vi "ObjectHandler.GetAllLogFiles.vi"(8 "error in (no error)":errorcluster, 11 "ObjectHandler in":refnum<class "ObjectHandler.lvclass">) -> (0 "error out":errorcluster, 1 "Found?":bool, 2 "Array":T1[](array[typedef]), 3 "ObjectHandler out":refnum<class "ObjectHandler.lvclass">)   [LabVIEW 2016, in "ObjectHandler.lvclass"]
uses:
  ObjectHandler.lvclass
  ObjectHandler.ObjectWType.ctl
  ObjectHandler.ObjectType.ctl
  ObjectHandler.lvclass/ObjectHandler.ctl
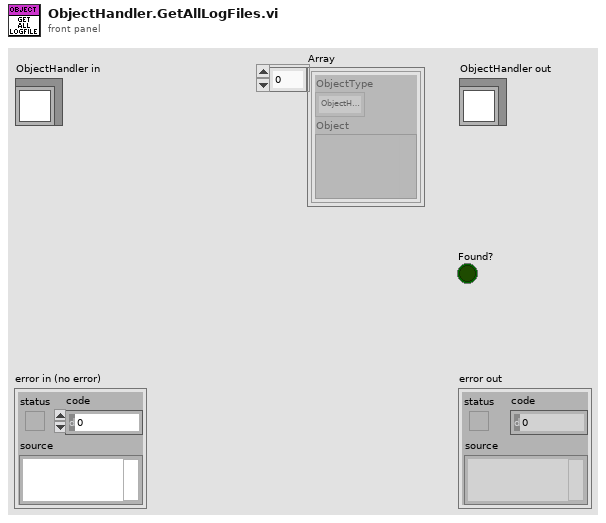
[diagram p1: front panel]
types:
  T1 = typedef "ObjectHandler.lvclass/ObjectHandler.ObjectWType.ctl" = cluster{"ObjectType":T2, "Object":variant}
  T2 = typedef "ObjectHandler.lvclass/ObjectHandler.ObjectType.ctl" = enum16{"undefined", "ObjectHandler", "ViHandler", "ErrorHandler", "CentralStorage", "Hausmodell", "Sondenmodell", "Wärmepumpe", "Umgebung"}
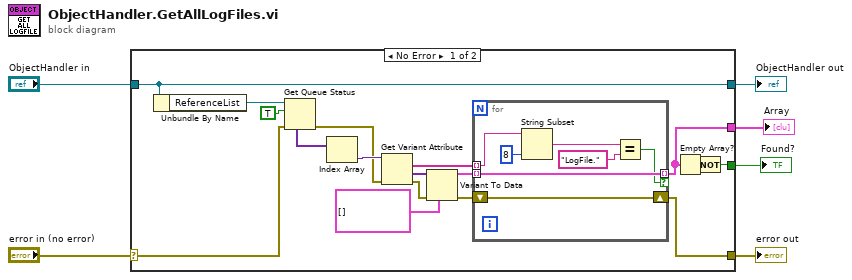
[diagram p0: block diagram]
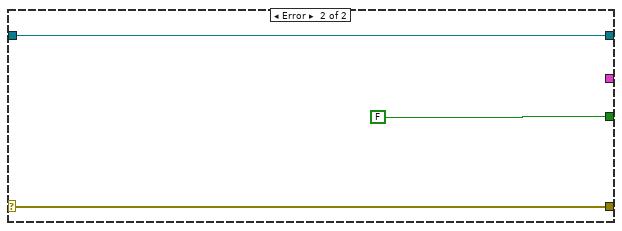
[diagram p2: hidden frame]
diagram:
  n1 = case shown="No Error" "error in (no error)" {
    selector: "error in (no error)" -> [w21 w32]
    tunnel: [w10 w32] -> w5
    tunnel: [w23 w33] -> w3
    tunnel: "ObjectHandler in" -> [w23 w33]
    tunnel: [w7 FALSE] -> w2
    tunnel: [w8 _] -> w1
    frame No Error {
      n2 = Unbundle By Name(w23) -> ("ReferenceList"=w22:refnum<queue>)
      n3 = Get Queue Status(queue=w22, return elements? (F)=TRUE, error in (no error)=w21) -> (error out=w17:errorcluster, elements=w20:variant[])  [unwired: 6 out]
      n4 = Index Array(array=w20) -> (element=w18:variant)  [unwired: 1 in]
      n5 = Get Variant Attribute(Variant=w18, error in=w17) -> (names=w11:string[], values=w16:variant[], error out=w14:errorcluster)  [unwired: 2 in, 1 out]
      n6 = Variant To Data(error in=w14, type=T1[] [] ("Array"), Variant=w16) -> (data=w12:T1[], error out=w13:errorcluster)
      n7 = for {
        shift-right: [w24] -> w10
        shift-left: w13 -> [w24]
        tunnel: w12 -> [w30] mode=indexing
        tunnel: w11 -> [w29] mode=indexing
        tunnel: [w30] -> w8 mode=indexing if=w25
        n8 = String Subset(string=w29, length (rest)=8 ("length (rest)")) -> (substring=w27:string)  [unwired: 1 in]
        n9 = Equal?(x=w27, y="LogFile." ("Name")) -> (x = y?=w25:bool)
      }
      n10 = Empty Array?(array=w8) -> (empty?=w9:bool)
      n11 = Not(x=w9) -> (.not. x?=w7:bool)
    }
    frame Error {
    }
  }
  "error out" <- w5
  "ObjectHandler out" <- w3
  "Array" <- w1
  "Found?" <- w2
